vi "Chs_to_Correlate.vi"(1 "Valid Ch to correlate":i32[](array[numeric])) -> (0 "Correlation Pairs":i32[][](array[numeric]))   [LabVIEW 2011]
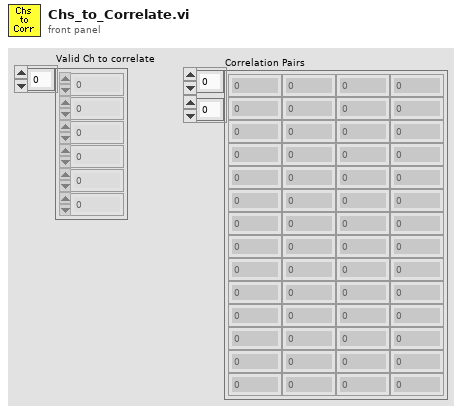
[diagram p1: front panel]
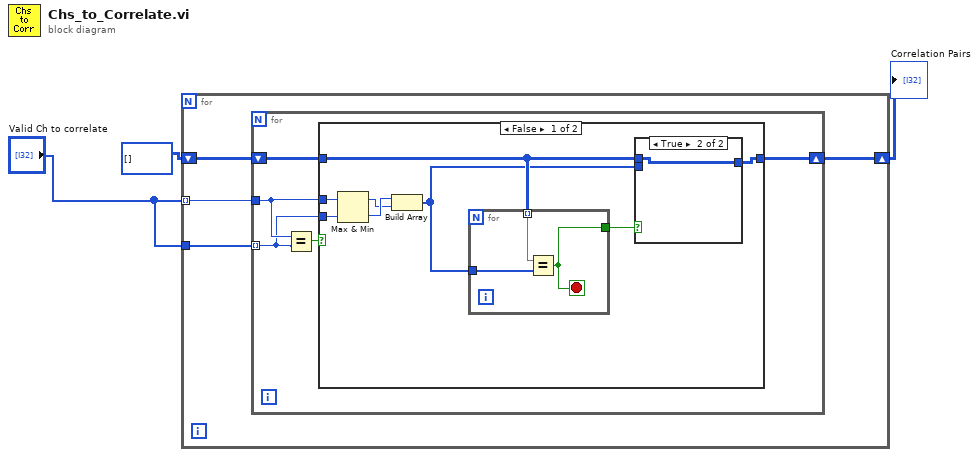
[diagram p0: block diagram]
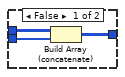
[diagram p2: hidden frame]
diagram:
  n1 = for {
    tunnel: "Valid Ch to correlate" -> [w7] mode=indexing
    tunnel: "Valid Ch to correlate" -> [w6]
    shift-right: [w5] -> w1
    shift-left: i32[][] [] -> [w4]
    n2 = for {
      tunnel: w7 -> [w10]
      tunnel: w6 -> [w8] mode=indexing
      shift-right: [w11] -> w5
      shift-left: w4 -> [w12]
      n3 = Equal?(x=w10, y=w8) -> (x = y?=w9:bool)
      n4 = case shown="False" w9 {
        tunnel: w12 -> [w15 w28]
        tunnel: [w16 w28] -> w11
        tunnel: w10 -> [w20 _]
        tunnel: w8 -> [w19 _]
        frame False {
          n5 = Max & Min(x=w20, y=w19) -> (max(x,y)=w17:i32, min(x,y)=w18:i32)
          n6 = Build Array(w18, w17) -> (w14:i32[])
          n7 = for {
            tunnel: w15 -> [w27] mode=indexing
            tunnel: w14 -> [w26]
            tunnel: [w25] -> w13
            stop <- w25 stop-if-true
            n8 = Equal?(x=w27, y=w26) -> (x = y?=w25:bool)
          }
          n9 = case shown="True" w13 {
            tunnel: [w23 w24] -> w16
            tunnel: w15 -> [w22 w24]
            tunnel: w14 -> [w21 _]
            frame False {
              n10 = Build Array (concatenate)(w22, w21) -> (w23:i32[][])
            }
            frame True {
            }
          }
        }
        frame True {
        }
      }
    }
  }
  "Correlation Pairs" <- w1
